vi "ManualControl.vi"() -> ()   [LabVIEW 2017]
panel:
  in  "manual control":T1
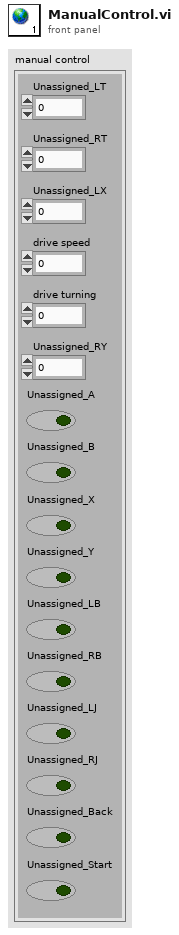
[diagram p1: front panel]
types:
  T1 = cluster{"drive speed":dbl, "drive turning":dbl, "Unassigned_LX":dbl, "Unassigned_RY":dbl, "Unassigned_A":bool, "Unassigned_RT":dbl, "Unassigned_LT":dbl, "Unassigned_B":bool, "Unassigned_X":bool, "Unassigned_Y":bool, "Unassigned_LB":bool, "Unassigned_RB":bool, "Unassigned_LJ":bool, "Unassigned_RJ":bool, "Unassigned_Back":bool, "Unassigned_Start":bool}
diagram:
